vi "GetIntFromRadioCtrl.vi"(11 "ref in":refnum<vi>) -> (2 "out":i32, 3 "ref out":refnum<vi>)   [LabVIEW 2018, in "Library-Ctrl.lvlib"]
uses:
  Library-Ctrl.lvlib
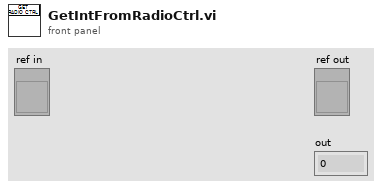
[diagram p1: front panel]
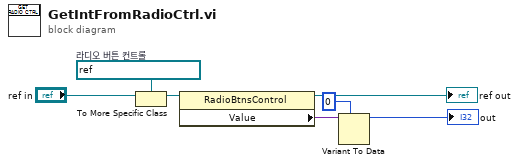
[diagram p0: block diagram]
diagram:
  w6 = refnum<vi> refnum  # 라디오 버튼 컨트롤
  n1 = To More Specific Class(target class=w6, reference="ref in") -> (specific class reference=w5:refnum<vi>)  [unwired: 1 in, 1 out]
  n2 = property class="RadioBtnsControl"(reference=w5) -> (reference out=→"ref out":refnum<vi>, "Value"=w4:variant)  [unwired: 1 in, 1 out]
  n3 = Variant To Data(type=0, Variant=w4) -> (data=→"out":i32)  [unwired: 1 in, 1 out]
